vi "Table cell - Set colour.vi"(8 "error in":errorcluster, 9 "Active Cell Background Color":u32(colorbox), 10 "Table Active Cell":T1, 11 "Table Reference":refnum<vi>) -> (0 "error out":errorcluster)   [LabVIEW 2011]
doc: "Set the background colour of a table cell specified by 'Table Active Cell'.\n\nInputs:\n Table Reference: Reference to a table.\n Table Active Cell: (x,y) position of the active cell.\n Active Cell Background colour: Integer representing the background colour of the defined active cell.\n Error in: Describes error conditions that occur before this node runs. This input provides standard error in functionality.\n\nOutputs:\n Error out: Contains error information. This output provides standard error out functionality."
uses:
  <vilib>/Utility/miscctls.llb/LVRowAndColumnTypeDef.ctl
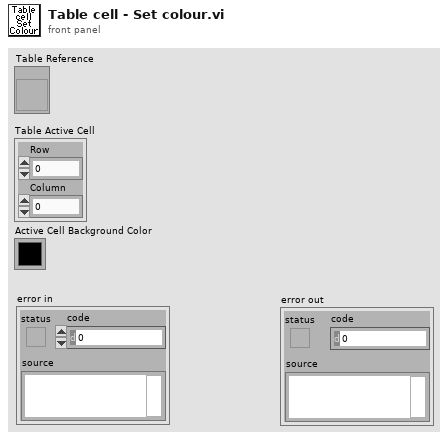
[diagram p1: front panel]
types:
  T1 = typedef "LVRowAndColumnTypeDef.ctl" = cluster{"Row":i32, "Column":i32}
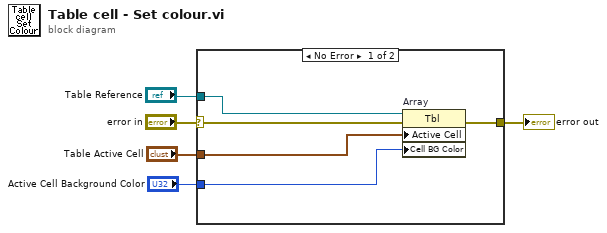
[diagram p0: block diagram]
diagram:
  n1 = case shown="No Error" "error in" {
    selector: "error in" -> [w7 w11]
    tunnel: "Table Reference" -> [w6 _]
    tunnel: [w10 w11] -> w5
    tunnel: "Table Active Cell" -> [w9 _]
    tunnel: "Active Cell Background Color" -> [w8 _]
    frame No Error {
      n2 = property on="Array" class="Tbl"(reference=w6, error in=w7, "Active Cell"=w9, "Cell BG Color"=w8) -> (error out=w10:errorcluster)  [unwired: 1 out]
    }
    frame Error {
    }
  }
  "error out" <- w5
